vi "Curtin1_Share.vi"(11 "Files":T1[](array[typedef])) -> ()   [LabVIEW 2022 SP3]
uses:
  Curtin1_Label.ctl
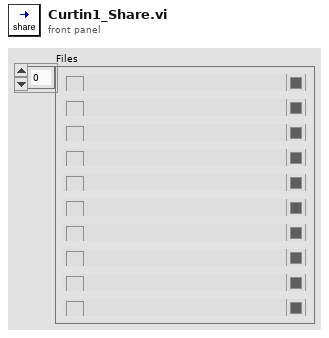
[diagram p1: front panel]
types:
  T1 = typedef "Curtin1_Label.ctl" = cluster{"Show?":bool, "Name":string, "Color":u32, "Path":path, "Show Notes":bool}
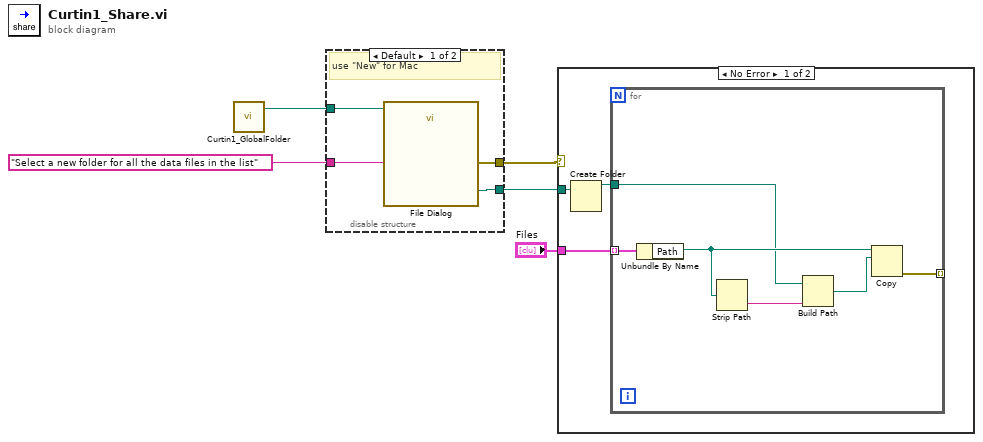
[diagram p0: block diagram]
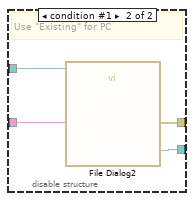
[diagram p2: hidden frame]
diagram:
  n1 = call "Curtin1_GlobalFolder.vi"() -> ("LabVIEW Data Path"=w1:path)  [unwired: 1 in, 1 out]
  n2 = disable-structure shown="Default" {
    disable-tunnel: [w9 w13] -> w4
    disable-tunnel: "Select a new folder for all the data files in the list" ("prompt") -> [w8 w12]
    disable-tunnel: [w7 w11] -> w2
    disable-tunnel: w1 -> [w6 w10]
    frame condition #0 (active) {
      # "use \"New\" for Mac"
      n3 = call "File Dialog"("start path"=w6, "prompt"=w8) -> ("selected path"=w9:path, "error out"=w7:errorcluster)  [unwired: 10 in, 2 out]
    }
    frame condition #1 {
      # "Use \"Existing\" for PC"
      n4 = call "File Dialog2"("start path"=w10, "prompt"=w12) -> ("selected path"=w13:path, "error out"=w11:errorcluster)  [unwired: 10 in, 2 out]
    }
  }
  n5 = case shown="No Error" w2 {
    tunnel: "Files" -> [w16 _]
    tunnel: w4 -> [w15 _]
    frame No Error {
      n6 = Create Folder(path (use dialog)=w15) -> (created path=w14:path)  [unwired: 2 in, 2 out]
      n7 = for {
        tunnel: w16 -> [w22] mode=indexing
        tunnel: w14 -> [w18]
        tunnel: [w17] -> _ mode=indexing
        n8 = Unbundle By Name(w22) -> ("Path"=w21:path)
        n9 = Strip Path(path=w21) -> (name=w20:string)  [unwired: 1 out]
        n10 = Build Path(base path=w18, name or relative path=w20) -> (appended path=w19:path)
        n11 = Copy(10:w19, 11:w21) -> (0:w17:errorcluster)  [unwired: 3 in, 2 out]
      }
    }
    frame Error {
    }
  }
